vi "IsConnected.vi"(8 "error in (no error)":errorcluster, 11 "NetworkStreamReader in":refnum<class "NetworkStreamReader.lvclass">) -> (0 "error out":errorcluster, 2 "Connected?":bool, 3 "NetworkStreamReader out":refnum<class "NetworkStreamReader.lvclass">)   [LabVIEW 2013, in "NetworkStreamReader.lvclass"]
doc: "Returns whether or not the NetworkStreamReader Object is currently connected to a corresponding NetworkStreamWriter across the network.\n\nJared Kirschner, 2012."
uses:
  NetworkStreamReader.lvclass
  NetworkStreamReader.lvclass/NetworkStreamReader.ctl
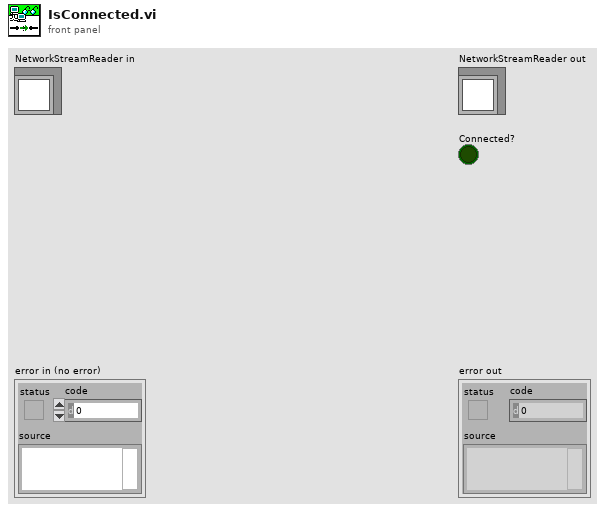
[diagram p1: front panel]
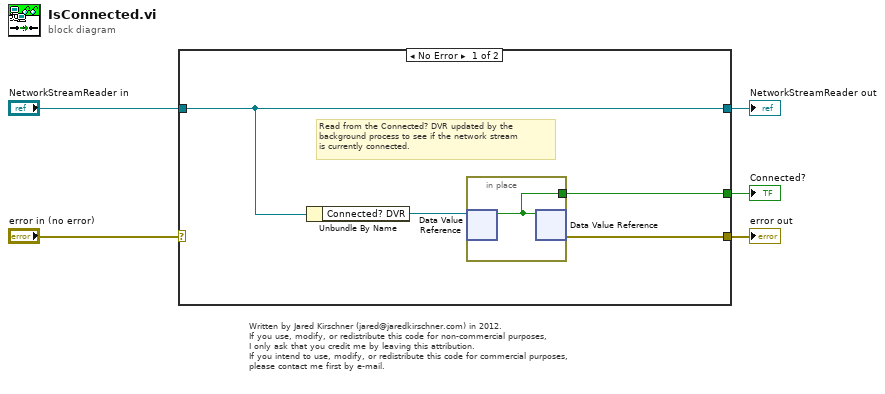
[diagram p0: block diagram]
diagram:
  # "Written by Jared Kirschner (jared@jaredkirschner.com) in 2012.\nIf you use, modify, or redistribute this code for non-commercial purposes,\nI only ask that you credit me by leaving this attribution.\nIf you intend to use, modify, or redistribute this code for commercial purposes,\nplease contact me first by e-mail."
  n1 = case shown="No Error" "error in (no error)" {
    selector: "error in (no error)" -> [_ w12]
    tunnel: [w7 w12] -> w4
    tunnel: [w8 w11] -> w2
    tunnel: "NetworkStreamReader in" -> [w8 w11]
    tunnel: [w6 _] -> w1
    frame No Error {
      # "Read from the Connected? DVR updated by the\nbackground process to see if the network stream\nis currently connected."
      n2 = Unbundle By Name(w8) -> ("Connected? DVR"=w9:refnum<data-value>)
      n3 = in-place {
        in-place-border: [w10] -> w6
        n4 = in-place-dvr #1(w9) -> (w10:bool)  [unwired: 1 out]
        n5 = in-place-dvr #1(w10) -> (w7:errorcluster)  [unwired: 1 out]
      }
    }
    frame Error {
    }
  }
  "error out" <- w4
  "NetworkStreamReader out" <- w2
  "Connected?" <- w1
